vi "PRLIDAR_5byte_Pasing.vi"(11 "RPLIDAR_Data":string) -> (0 "Distance(mm)":dbl[](array[numeric]), 3 "Theta(deg)":dbl[](array[numeric]))   [LabVIEW 2024]
panel:
  out "숫자형":i32
  out "C 배열":u8[](array[numeric])
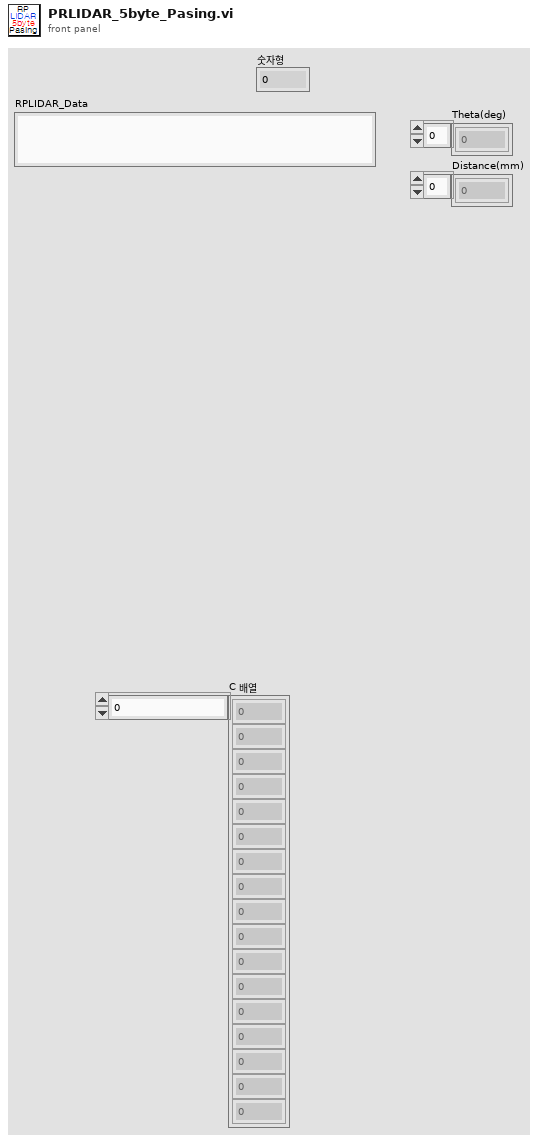
[diagram p1: front panel]
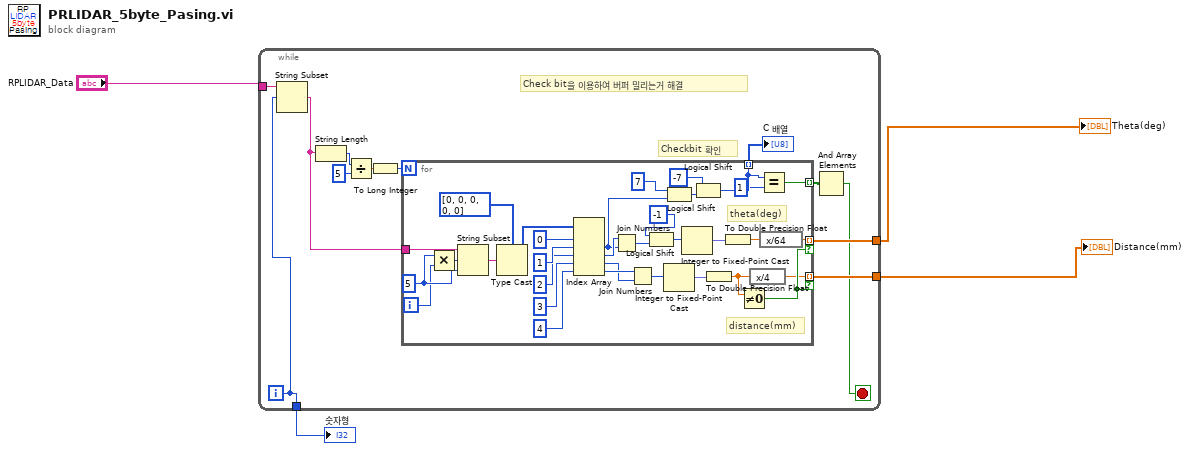
[diagram p0: block diagram]
diagram:
  n1 = while {
    tunnel: [w16] -> w2
    tunnel: [w15] -> w1
    tunnel: "RPLIDAR_Data" -> [w9]
    tunnel: [w5] -> w4
    i -> [w5]
    stop <- w6 stop-if-true
    # "Check bit을 이용하여 버퍼 밀리는거 해결"
    # "Checkbit 확인"
    n2 = String Subset(string=w9, offset (0)=w5) -> (substring=w8:string)  [unwired: 1 in]
    n3 = String Length(string=w8) -> (length=w10:i32)
    n4 = Divide(x=w10, y=5) -> (x/y=w12:dbl)
    n5 = To Long Integer(number=w12) -> (32bit integer=w11:i32)
    n6 = for {
      N: w11 -> [_]
      tunnel: [w26] -> w16 mode=indexing if=w38
      tunnel: [w25] -> w15 mode=indexing if=w38
      tunnel: w8 -> [w36]
      tunnel: [w19] -> w14 mode=indexing
      tunnel: [w17] -> w7 mode=indexing
      i -> [w40]
      w41 = 5 ("x")
      # "theta(deg)"
      # "distance(mm)"
      n7 = Multiply(x=w41, y=w40) -> (x*y=w29:i32)
      n8 = String Subset(string=w36, offset (0)=w29, length (rest)=w41) -> (substring=w28:string)
      n9 = Type Cast(type=u8[] [0, 0, 0, 0, 0], x=w28) -> (*(type *) &x=w27:u8[])
      n10 = Index Array(array=w27, index #1=0 ("index"), index #2=1 ("index"), index #3=2 ("index"), index #4=3 ("index"), index #5=4 ("index")) -> (element #2=w20:u8, element #3=w43:u8, element #4=w37:u8, element #5=w44:u8)  [unwired: 1 out]
      n11 = Join Numbers(hi=w43, lo=w20) -> ((hi.lo)=w24:u16)
      n12 = Join Numbers(hi=w44, lo=w37) -> ((hi.lo)=w42:u16)
      n13 = Logical Shift(y=i16 -1, x=w24) -> (x << y=w31:u16)
      n14 = Logical Shift(y=i16 7, x=w20) -> (x << y=w22:u8)
      n15 = Integer to Fixed-Point Cast(integer=w42) -> (fixed-point=w34:fxp<+,16,16>)  [unwired: 1 in]
      n16 = Integer to Fixed-Point Cast(integer=w31) -> (fixed-point=w35:fxp<+,16,16>)  [unwired: 1 in]
      n17 = Logical Shift(y=i16 -7, x=w22) -> (x << y=w19:u8)
      n18 = To Double Precision Float(number=w34) -> (double precision float=w33:dbl)
      n19 = To Double Precision Float(number=w35) -> (double precision float=w32:dbl)
      n20 = Not Equal To 0?(x=w33) -> (x != 0?=w38:bool)
      n21 = expression code="x/4"(w33) -> (w25:dbl)
      n22 = Equal?(x=w19, y=u8 1) -> (x = y?=w17:bool)
      n23 = expression code="x/64"(w32) -> (w26:dbl)
    }
    "C 배열" <- w14
    n24 = And Array Elements(Boolean array=w7) -> (logical AND=w6:bool)
  }
  "Theta(deg)" <- w2
  "Distance(mm)" <- w1
  "숫자형" <- w4
